vi "Read Selected TDMS File.vi"(8 "error in (no error)":errorcluster, 11 "TDMS Data Source in":refnum<class "TDMS Data Source.lvclass">) -> (0 "error out":errorcluster, 2 "Selected TDMS File":path caption="start path", 3 "TDMS Data Source out":refnum<class "TDMS Data Source.lvclass">)   [LabVIEW 2020, in "TDMS Data Source.lvlib" / "TDMS Data Source.lvclass"]
uses:
  TDMS Data Source.lvclass
  TDMS Data Source.lvclass/TDMS Data Source.ctl
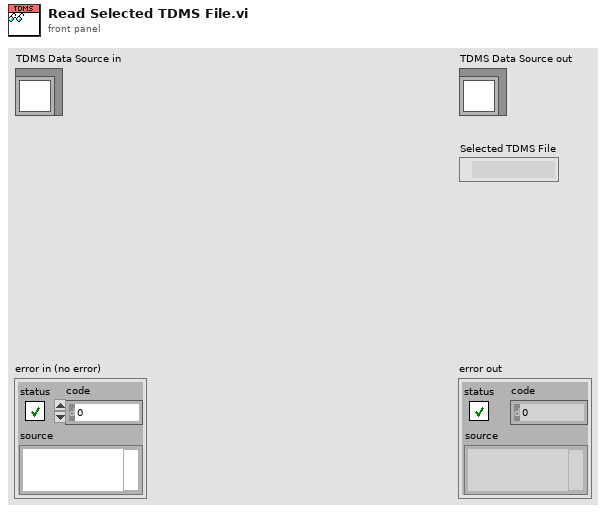
[diagram p1: front panel]
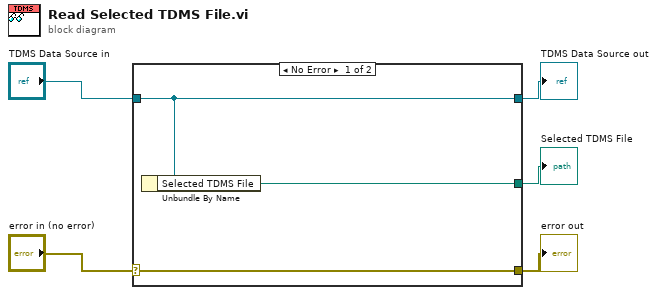
[diagram p0: block diagram]
diagram:
  n1 = case shown="No Error" "error in (no error)" {
    selector: "error in (no error)" -> [w8 w9]
    tunnel: [w8 w9] -> w4
    tunnel: [w7 w10] -> w2
    tunnel: "TDMS Data Source in" -> [w7 w10]
    tunnel: [w6 _] -> w1
    frame No Error {
      n2 = Unbundle By Name(w7) -> ("Selected TDMS File"=w6:path)
    }
    frame Error {
    }
  }
  "error out" <- w4
  "TDMS Data Source out" <- w2
  "Selected TDMS File" <- w1
